vi "Logger.Variant.Write.vi"(8 "error in (no error)":errorcluster, 10 "VariantSets":T1={"State"=enum."Init", "ImgPath"=path "", "WabcoPlate"="", "WabcoProduct"="", "ClientProduct"="", "ClientPlate"="", "TotalQuantity"=0, "OrderQuantity"=0, "Serial"=0, "Wabco"={"LaserJob"="", "AdditionalTxt"="037", "FactoryCode"="", "RevID"=0, "ForkID"=0, "FailuresLimit"=0, "GlobalCnt"=0, "ScannerProgram"=0, "SerialFormat"=enum."6 dig", "CoordA"={"X"=0.0, "Y"=0.0, "Angle"=0.0}, "CoordB"={"X"=0.0, "Y"=0.0, "Angle"=0.0}, "DMCconfig"=0}, "Client"={"LaserJob"="", "AdditionalTxt"="", "FactoryCode"="037", "RevID"=0, "ForkID"=0, "FailuresLimit"=0, "GlobalCnt"=0, "ScannerProgram"=0, "SerialFormat"=enum."6 dig", "CoordA"={"X"=0.0, "Y"=0.0, "Angle"=0.0}, "CoordB"={"X"=0.0, "Y"=0.0, "Angle"=0.0}, "DMCconfig"=0}}) -> (0 "error out":errorcluster)   [LabVIEW 2016]
uses:
  Logger.Variant.Sets.ctl
  Station/Station.Changeover.State.vi
  Station/Station.Plate.Properties.ctl
  Sequence/Sequence.Code.SerialFormat.ctl
  Drivers/V7310/LowLevel/V7310.Job.Sets.ctl
  Global/ApplicationGlobal.vi
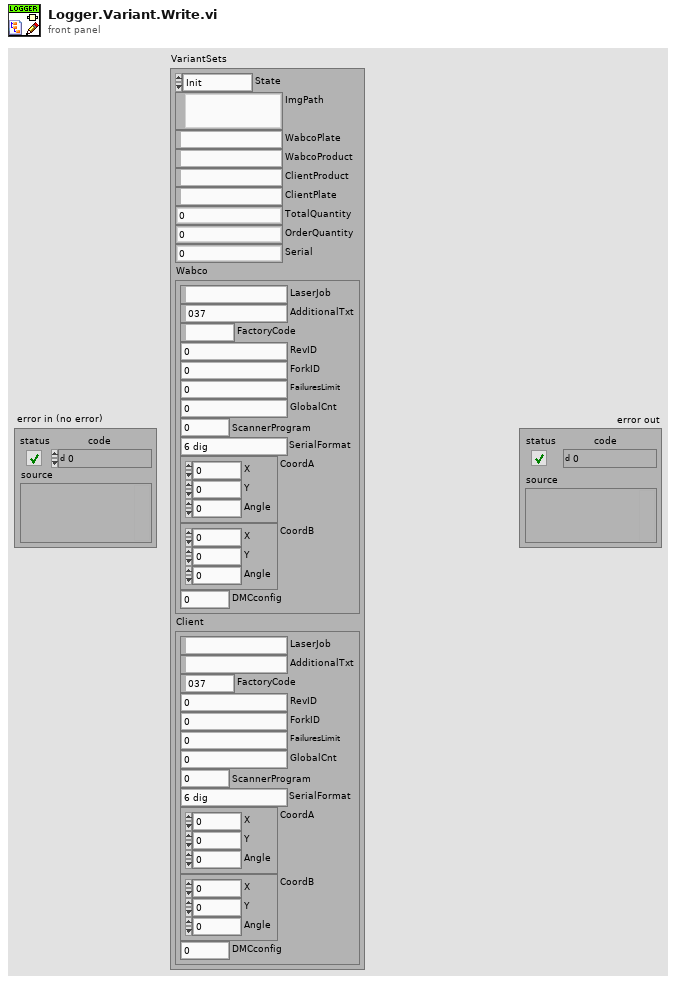
[diagram p1: front panel]
types:
  T1 = typedef "Logger.Variant.Sets.ctl" = cluster{"State":T2, "ImgPath":path, "WabcoPlate":string, "WabcoProduct":string, "ClientProduct":string, "ClientPlate":string, "TotalQuantity":u16, "OrderQuantity":u16, "Serial":i32, "Wabco":T3, "Client":T3}
  T2 = typedef "Station.Changeover.State.vi" = enum16{"Init", "Scaning", "NOK", "Wait for ack", "Ready"}
  T3 = typedef "Station.Plate.Properties.ctl" = cluster{"LaserJob":string, "AdditionalTxt":string, "FactoryCode":string, "RevID":u8, "ForkID":u8, "FailuresLimit":u16, "GlobalCnt":i32, "ScannerProgram":u8, "SerialFormat":T4, "CoordA":T5, "CoordB":T5, "DMCconfig":i32}
  T4 = typedef "Sequence.Code.SerialFormat.ctl" = enum8{"", "6 dig", "7 dig"}
  T5 = typedef "V7310.Job.Sets.ctl" = cluster{"X":dbl, "Y":dbl, "Angle":dbl}
  T6 = cluster{"WabcoPlate":string, "WabcoProduct":string, "ClientProduct":string, "ClientPlate":string}
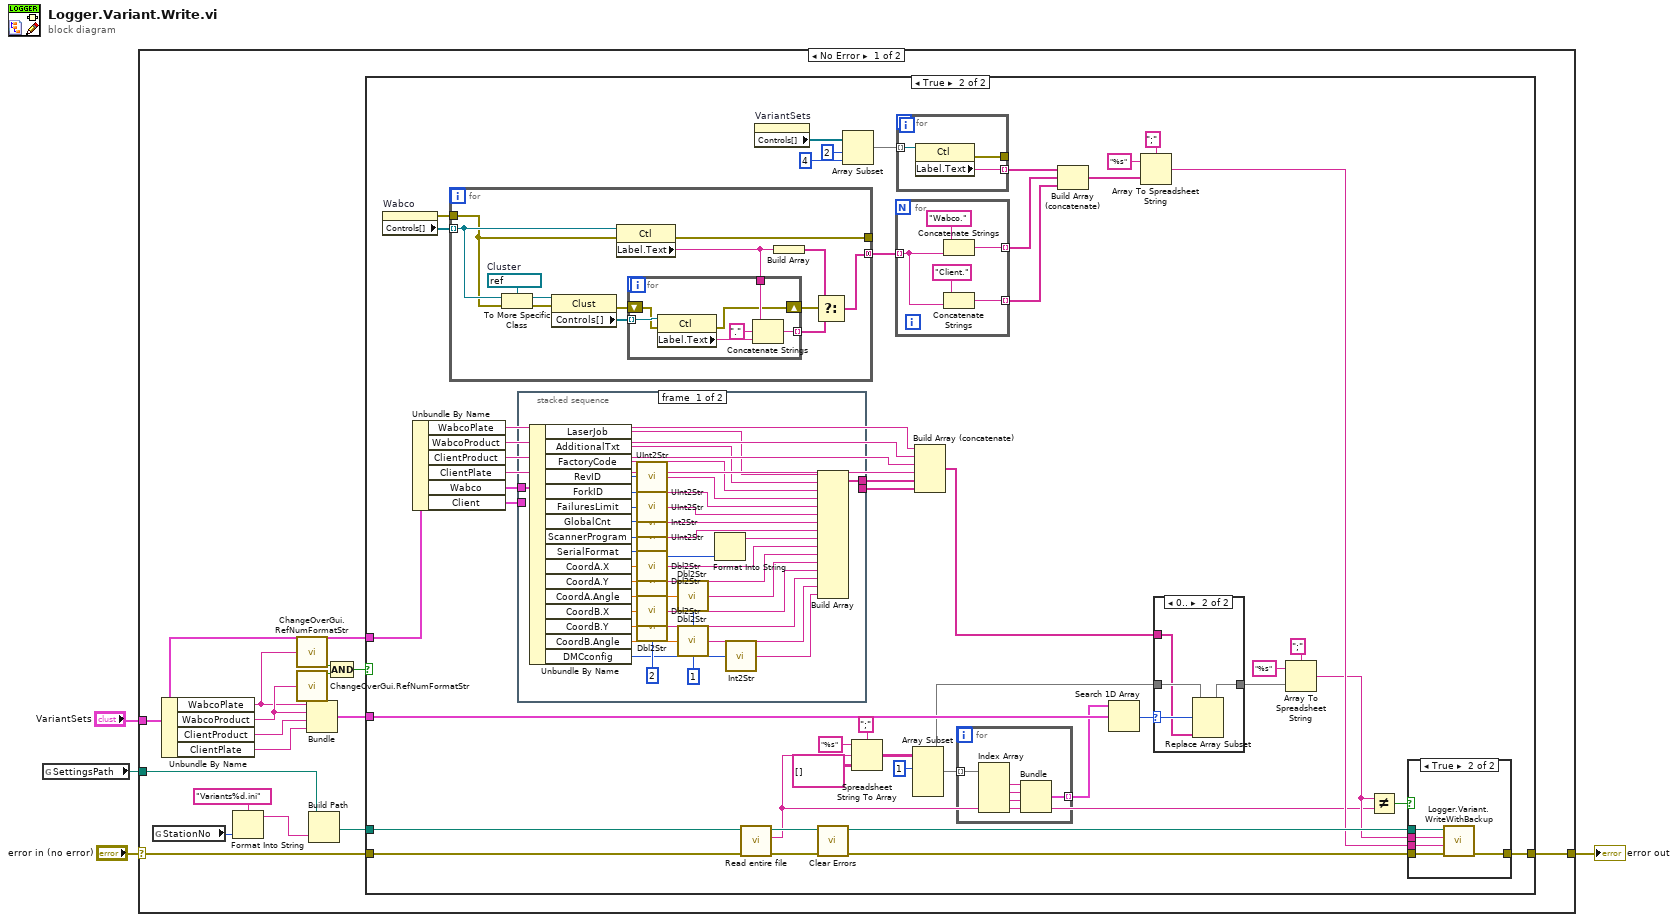
[diagram p0: block diagram]
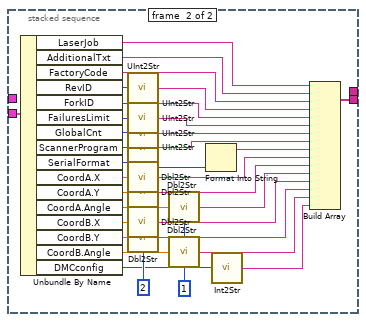
[diagram p4: hidden frame]
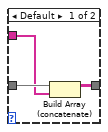
[diagram p5: hidden frame]
diagram:
  n1 = global read "ApplicationGlobal.vi" "SettingsPath"() -> (w2:path)
  n2 = case shown="No Error" "error in (no error)" {
    selector: "error in (no error)" -> [w20 w179]
    tunnel: [w19 w179] -> w3
    tunnel: w2 -> [w8 _]
    tunnel: "VariantSets" -> [w10 _]
    frame No Error {
      n3 = global read "ApplicationGlobal.vi" "StationNo"() -> (w5:i32)
      n4 = Unbundle By Name(w10) -> ("WabcoPlate"=w15:string, "WabcoProduct"=w16:string, "ClientProduct"=w17:string, "ClientPlate"=w9:string)
      n5 = Format Into String(format string="Variants%d.ini", w5) -> (resulting string=w6:string)  [unwired: 2 in, 1 out]
      n6 = call "ChangeOverGui.RefNumFormatStr.vi"("RefNum in"=w15) -> ("RefNum format ok?"=w14:bool)  [unwired: 2 out]
      n7 = call "ChangeOverGui.RefNumFormatStr.vi"("RefNum in"=w16) -> ("RefNum format ok?"=w13:bool)  [unwired: 2 out]
      n8 = Bundle("WabcoPlate"=w15, "WabcoProduct"=w16, "ClientProduct"=w17, "ClientPlate"=w9) -> (w11:T6)  [unwired: 1 in]
      n9 = Build Path(base path=w8, name or relative path=w6) -> (appended path=w18:path)
      n10 = Compound Arithmetic op=AND(w14, w13) -> (w12:bool)
      n11 = case shown="True" w12 {
        tunnel: w20 -> [w21 w65]
        tunnel: [w21 w56] -> w19
        tunnel: w18 -> [_ w51]
        tunnel: w11 -> [_ w60]
        tunnel: w10 -> [_ w44]
        frame False {
        }
        frame True {
          n12 = property on="Wabco" class="Clust (strict)"() -> (error out=w26:errorcluster, "Controls[]"=w27:refnum<vi>[])  [unwired: 2 in, 1 out]
          n13 = Unbundle By Name(w44) -> ("WabcoPlate"=w34:string, "WabcoProduct"=w33:string, "ClientProduct"=w32:string, "ClientPlate"=w31:string, "Wabco"=w40:T3, "Client"=w37:T3)
          n14 = for {
            tunnel: w27 -> [w85] mode=indexing
            tunnel: [w78] -> w30 mode=concatenating
            tunnel: [w89] -> _
            tunnel: w26 -> [w77]
            w87 = refnum<vi> refnum  # Cluster
            n15 = To More Specific Class(target class=w87, reference=w85, error in=w77) -> (specific class reference=w86:refnum<vi>, error out=w88:errorcluster)
            n16 = property class="Clust"(reference=w86, error in=w88) -> (error out=w83:errorcluster, "Controls[]"=w84:refnum<vi>[])  [unwired: 1 out]
            n17 = property class="Ctl"(reference=w85, error in=w77) -> (error out=w89:errorcluster, "Label.Text"=w82:string)  [unwired: 1 out]
            n18 = for {
              tunnel: w84 -> [w96] mode=indexing
              tunnel: [w93] -> w79 mode=indexing
              tunnel: w82 -> [w92]
              shift-right: [w90] -> w81
              shift-left: w83 -> [w95]
              n19 = property class="Ctl"(reference=w96, error in=w95) -> (error out=w90:errorcluster, "Label.Text"=w94:string)  [unwired: 1 out]
              n20 = Concatenate Strings(w92, "." ("string"), w94) -> (w93:string)
            }
            n21 = Build Array(w82) -> (w80:string[])
            n22 = Select(t=w80, s=w81, f=w79) -> (s? t:f=w78:string[])
          }
          n23 = stacked-sequence {
            tunnel: w40 -> [w129 _]
            tunnel: [w101 _] -> w39
            tunnel: [_ w135] -> w38
            tunnel: w37 -> [_ w134]
            frame #0 {
              w127 = i16 2 ("precision (6)")
              w128 = i16 1 ("precision (6)")
              n24 = Unbundle By Name(w129) -> ("LaserJob"=w102:string, "AdditionalTxt"=w103:string, "FactoryCode"=w104:string, "RevID"=w111:u8, "ForkID"=w112:u8, "FailuresLimit"=w110:u16, "GlobalCnt"=w109:i32, "ScannerProgram"=w98:u8, "SerialFormat"=w114:T4, "CoordA.X"=w126:dbl, "CoordA.Y"=w125:dbl, "CoordA.Angle"=w124:dbl, "CoordB.X"=w123:dbl, "CoordB.Y"=w122:dbl, "CoordB.Angle"=w121:dbl, "DMCconfig"=w100:i32)
              n25 = call "UInt2Str.vi"("Numeric"=w111) -> ("string"=w105:string)
              n26 = call "UInt2Str.vi"("Numeric"=w112) -> ("string"=w106:string)
              n27 = call "UInt2Str.vi"("Numeric"=w110) -> ("string"=w107:string)
              n28 = call "Int2Str.vi"("Numeric"=w109) -> ("string"=w108:string)
              n29 = call "UInt2Str.vi"("Numeric"=w98) -> ("string"=w97:string)
              n30 = call "Dbl2Str.vi"("Numeric"=w126, "precision (6)"=w127) -> ("string"=w115:string)
              n31 = call "Dbl2Str.vi"("Numeric"=w125, "precision (6)"=w127) -> ("string"=w116:string)
              n32 = call "Dbl2Str.vi"("Numeric"=w123, "precision (6)"=w127) -> ("string"=w118:string)
              n33 = call "Dbl2Str.vi"("Numeric"=w122, "precision (6)"=w127) -> ("string"=w119:string)
              n34 = call "Dbl2Str.vi"("Numeric"=w124, "precision (6)"=w128) -> ("string"=w117:string)
              n35 = call "Dbl2Str.vi"("Numeric"=w121, "precision (6)"=w128) -> ("string"=w120:string)
              n36 = Format Into String(w114) -> (resulting string=w113:string)  [unwired: 3 in, 1 out]
              n37 = call "Int2Str.vi"("Numeric"=w100) -> ("string"=w99:string)
              n38 = Build Array(w102, w103, w104, w105, w106, w107, w108, w97, w113, w115, w116, w117, w118, w119, w120, w99) -> (w101:string[])
            }
            frame #1 {
              w161 = i16 2 ("precision (6)")
              w162 = i16 1 ("precision (6)")
              n39 = Unbundle By Name(w134) -> ("LaserJob"=w136:string, "AdditionalTxt"=w137:string, "FactoryCode"=w138:string, "RevID"=w145:u8, "ForkID"=w146:u8, "FailuresLimit"=w144:u16, "GlobalCnt"=w143:i32, "ScannerProgram"=w131:u8, "SerialFormat"=w148:T4, "CoordA.X"=w160:dbl, "CoordA.Y"=w159:dbl, "CoordA.Angle"=w158:dbl, "CoordB.X"=w157:dbl, "CoordB.Y"=w156:dbl, "CoordB.Angle"=w155:dbl, "DMCconfig"=w133:i32)
              n40 = call "UInt2Str.vi"("Numeric"=w145) -> ("string"=w139:string)
              n41 = call "UInt2Str.vi"("Numeric"=w146) -> ("string"=w140:string)
              n42 = call "UInt2Str.vi"("Numeric"=w144) -> ("string"=w141:string)
              n43 = call "UInt2Str.vi"("Numeric"=w143) -> ("string"=w142:string)
              n44 = call "UInt2Str.vi"("Numeric"=w131) -> ("string"=w130:string)
              n45 = call "Dbl2Str.vi"("Numeric"=w160, "precision (6)"=w161) -> ("string"=w149:string)
              n46 = call "Dbl2Str.vi"("Numeric"=w159, "precision (6)"=w161) -> ("string"=w150:string)
              n47 = call "Dbl2Str.vi"("Numeric"=w157, "precision (6)"=w161) -> ("string"=w152:string)
              n48 = call "Dbl2Str.vi"("Numeric"=w156, "precision (6)"=w161) -> ("string"=w153:string)
              n49 = call "Dbl2Str.vi"("Numeric"=w158, "precision (6)"=w162) -> ("string"=w151:string)
              n50 = call "Dbl2Str.vi"("Numeric"=w155, "precision (6)"=w162) -> ("string"=w154:string)
              n51 = Format Into String(w148) -> (resulting string=w147:string)  [unwired: 3 in, 1 out]
              n52 = call "Int2Str.vi"("Numeric"=w133) -> ("string"=w132:string)
              n53 = Build Array(w136, w137, w138, w139, w140, w141, w142, w130, w147, w149, w150, w151, w152, w153, w154, w132) -> (w135:string[])
            }
          }
          n54 = call "Read entire file.vi"("error in"=w65, "file"=w51) -> ("error out"=w55:errorcluster, "contents"=w23:string)  [unwired: 4 in]
          n55 = property on="VariantSets" class="Clust (strict)"() -> ("Controls[]"=w42:refnum<vi>[])  [unwired: 2 in, 2 out]
          n56 = call <vilib>:"Clear Errors.vi"("error in (no error)"=w55) -> ("error out"=w47:errorcluster)  [unwired: 5 in, 1 out]
          n57 = Array Subset(array=w42, index=2, length=4) -> (w36:refnum<vi>[])
          n58 = Spreadsheet String To Array(delimiter (Tab)=";", format string="%s", spreadsheet string=w23, array type (2D Dbl)=string[][] []) -> (array=w57:string[][])
          n59 = for {
            tunnel: w30 -> [w73] mode=indexing
            tunnel: [w75] -> w29 mode=indexing
            tunnel: [w72] -> w28 mode=indexing
            n60 = Concatenate Strings("Wabco." ("string"), w73) -> (w75:string)
            n61 = Concatenate Strings("Client." ("string"), w73) -> (w72:string)
          }
          n62 = for {
            tunnel: w36 -> [w178] mode=indexing
            tunnel: [w177] -> w48 mode=indexing
            tunnel: [w176] -> _
            n63 = property class="Ctl"(reference=w178) -> (error out=w176:errorcluster, "Label.Text"=w177:string)  [unwired: 1 in, 1 out]
          }
          n64 = Array Subset(array=w57, index (row)=1 ("index")) -> (w46:string[][])  [unwired: 3 in]
          n65 = Build Array (concatenate)(w34, w33, w32, w31, w39, w38) -> (w41:string[])
          n66 = for {
            tunnel: w46 -> [w164] mode=indexing
            tunnel: [w165] -> w59 mode=indexing
            n67 = Index Array(array=w164) -> (element #1=w168:string, element #2=w167:string, element #3=w166:string, element #4=w163:string)  [unwired: 4 in]
            n68 = Bundle(w168, w167, w166, w163) -> (w165:cluster{string, string, string, string})  [unwired: 1 in]
          }
          n69 = Build Array (concatenate)(w48, w29, w28) -> (w35:string[])
          n70 = Search 1D Array(1D array=w59, element=w60) -> (index of element=w58:i32)  [unwired: 1 in]
          n71 = Array To Spreadsheet String(delimiter (Tab)=";", array=w35, 3:"%s" ("format string")) -> (spreadsheet string=w25:string)
          n72 = case shown="0.." w58 {
            selector: w58 -> [_ w173]
            tunnel: w46 -> [w171 w175]
            tunnel: [w169 w174] -> w54
            tunnel: w41 -> [w170 w172]
            frame Default {
              n73 = Build Array (concatenate)(w171, w170) -> (w169:string[][])
            }
            frame 0.. {
              n74 = Replace Array Subset(array=w175, new element=w172, index (row)=w173) -> (w174:string[][])  [unwired: 1 in]
            }
          }
          n75 = Array To Spreadsheet String(delimiter (Tab)=";", array=w54, 3:"%s" ("format string")) -> (spreadsheet string=w24:string)
          n76 = Not Equal?(x=w24, y=w23) -> (x != y?=w22:bool)
          n77 = case shown="True" w22 {
            tunnel: [w66 w71] -> w56
            tunnel: w51 -> [_ w70]
            tunnel: w47 -> [w66 w69]
            tunnel: w25 -> [_ w68]
            tunnel: w24 -> [_ w67]
            frame False {
            }
            frame True {
              n78 = call "Logger.Variant.WriteWithBackup.vi"("error in"=w69, "header"=w68, "addition"=w67, "file"=w70) -> ("error out"=w71:errorcluster)  [unwired: 7 in]
            }
          }
        }
      }
    }
    frame Error {
    }
  }
  "error out" <- w3
